vi "DSF.Engine.Memory.Buffer.Insert Channels.Preserve Value.vi"(8 "error in (no error)":errorcluster, 9 "Channel Configuration":T1 {"count" format="%d elements"; "offset" format="%d bytes"}, 10 "VS Channels Array in":dbl[](array[numeric]), 11 "Buffer in":refnum<class "DSF.Engine.Memory.Buffer.lvclass">) -> (0 "error out":errorcluster, 2 "VS Channels Array out":dbl[](array[numeric]), 3 "Buffer out":refnum<class "DSF.Engine.Memory.Buffer.lvclass">)   [LabVIEW 2016, in "DSF.Engine.lvlib" / "DSF.Engine.Memory.Buffer.lvclass"]
uses:
  DSF.Engine.Memory.Buffer.lvclass
  C:/Git/SourceTree/DSF/Source/Submodules/Memory Manager/Source/Classes/Pointer/Memory.Pointer.lvclass
  Typedefs/DSF.Engine.Buffer Channel Configuration.ctl
  Typedefs/DSF.Shared.Data Type.ctl
  Submodules/Memory Manager/Source/Classes/Pointer/Memory.Pointer.lvclass/Memory.Pointer.ctl
  DSF.Engine.Memory.Buffer.Write.1D.Bool.vi
  DSF.Engine.Memory.Buffer.Write.1D.SGL.vi
  DSF.Engine.Memory.Buffer.Write.1D.DBL.vi
  DSF.Engine.Memory.Buffer.Write.1D.I8.vi
  DSF.Engine.Memory.Buffer.Write.1D.I16.vi
  DSF.Engine.Memory.Buffer.Write.1D.I32.vi
  DSF.Engine.Memory.Buffer.Write.1D.I64.vi
  DSF.Engine.Memory.Buffer.Write.1D.U8.vi
  DSF.Engine.Memory.Buffer.Write.1D.U16.vi
  DSF.Engine.Memory.Buffer.Write.1D.U32.vi
  DSF.Engine.Memory.Buffer.Write.1D.U64.vi
  Submodules/Memory Manager/Source/Classes/Pointer/Methods/Memory.Pointer.Write.vi
  Submodules/Memory Manager/Source/Classes/Pointer/Methods/Memory.Pointer.Write.Safe.1D.Bool.vi
  Submodules/Memory Manager/Source/Classes/Pointer/Methods/Memory.Pointer.Write.Safe.1D.SGL.vi
  Submodules/Memory Manager/Source/Classes/Pointer/Methods/Memory.Pointer.Write.Safe.1D.DBL.vi
  Submodules/Memory Manager/Source/Classes/Pointer/Methods/Memory.Pointer.Write.Safe.1D.I8.vi
  Submodules/Memory Manager/Source/Classes/Pointer/Methods/Memory.Pointer.Write.Safe.1D.I16.vi
  Submodules/Memory Manager/Source/Classes/Pointer/Methods/Memory.Pointer.Write.Safe.1D.I32.vi
  Submodules/Memory Manager/Source/Classes/Pointer/Methods/Memory.Pointer.Write.Safe.1D.I64.vi
  Submodules/Memory Manager/Source/Classes/Pointer/Methods/Memory.Pointer.Write.Safe.1D.U8.vi
  Submodules/Memory Manager/Source/Classes/Pointer/Methods/Memory.Pointer.Write.Safe.1D.U16.vi
  Submodules/Memory Manager/Source/Classes/Pointer/Methods/Memory.Pointer.Write.Safe.1D.U32.vi
  Submodules/Memory Manager/Source/Classes/Pointer/Methods/Memory.Pointer.Write.Safe.1D.U64.vi
  Submodules/Memory Manager/Source/Classes/Pointer/Methods/Memory.Pointer.Write.Unsafe.1D.Bool.vi
  Submodules/Memory Manager/Source/Classes/Pointer/Methods/Memory.Pointer.Parameter Check.Null Pointer.vi
  Submodules/Memory Manager/Source/Classes/Pointer/Methods/Memory.Pointer.Parameter Check.Subset.Power of 2.vi
  Submodules/Memory Manager/Source/Classes/Pointer/Methods/Memory.Pointer.Write.Unsafe.1D.SGL.vi
  Submodules/Memory Manager/Source/Classes/Pointer/Methods/Memory.Pointer.Write.Unsafe.1D.DBL.vi
  Submodules/Memory Manager/Source/Classes/Pointer/Methods/Memory.Pointer.Write.Unsafe.1D.I8.vi
  Submodules/Memory Manager/Source/Classes/Pointer/Methods/Memory.Pointer.Write.Unsafe.1D.I16.vi
  Submodules/Memory Manager/Source/Classes/Pointer/Methods/Memory.Pointer.Write.Unsafe.1D.I32.vi
  Submodules/Memory Manager/Source/Classes/Pointer/Methods/Memory.Pointer.Write.Unsafe.1D.I64.vi
  Submodules/Memory Manager/Source/Classes/Pointer/Methods/Memory.Pointer.Write.Unsafe.1D.U8.vi
  Submodules/Memory Manager/Source/Classes/Pointer/Methods/Memory.Pointer.Write.Unsafe.1D.U16.vi
  Submodules/Memory Manager/Source/Classes/Pointer/Methods/Memory.Pointer.Write.Unsafe.1D.U32.vi
  Submodules/Memory Manager/Source/Classes/Pointer/Methods/Memory.Pointer.Write.Unsafe.1D.U64.vi
  Submodules/Memory Manager/Source/Classes/Pointer/Accessors/Get Address.vi
  Submodules/Memory Manager/Source/Classes/Pointer/Methods/Memory.Pointer.Errors.vi
  Submodules/Memory Manager/Source/Classes/Pointer/Methods/Memory.Pointer.Errors.Null Pointer.vi
  Submodules/Memory Manager/Source/Classes/Pointer/Methods/Memory.Pointer.Errors.Out of Bounds.vi
  Submodules/Memory Manager/Source/Classes/Pointer/Accessors/Get Size.vi
  Submodules/Memory Manager/Source/VIs/Memory.Count to Size.Power of 2.vi
  Submodules/Memory Manager/Source/Classes/Pointer/Methods/Memory.Pointer.Errors.Create Error.vi
  Submodules/Memory Manager/Source/Submodules/SEH/Source/VIs/Static Error Handling.Source Buffer.Write.String.vi
  Submodules/Memory Manager/Source/Classes/Pointer/Methods/Memory.Pointer.Errors.Write Pointer Size.vi
  Submodules/Memory Manager/Source/Submodules/SEH/Source/VIs/Static Error Handling.Source Buffer.Write.Numeric.Scalar.Base10.vi
  Submodules/Memory Manager/Source/Submodules/SEH/Source/VIs/Static Error Handling.Source Buffer.Write.Numeric.Scalar.Base10 (U64).vi
  Submodules/Memory Manager/Source/Submodules/SEH/Source/VIs/Static Error Handling.Error Cluster Constant.vi
  Submodules/Memory Manager/Source/Submodules/SEH/Source/VIs/Static Error Handling.Error Cluster Constant (256B).vi
  Submodules/Memory Manager/Source/Submodules/SEH/Source/VIs/Static Error Handling.Parameters.Status.Set.vi
  Submodules/Memory Manager/Source/Submodules/SEH/Source/VIs/Static Error Handling.Parameters.Code.Set.vi
  Submodules/Memory Manager/Source/Submodules/SEH/Source/VIs/Static Error Handling.Parameters.VI Source.Set.vi
  Submodules/Memory Manager/Source/Constants/Memory.Constants.vi
  Submodules/Memory Manager/Source/Constants/Memory.Constants.Library Name.vi
  Submodules/Memory Manager/Source/Classes/Pointer/Methods/Memory.Pointer.Errors.Get Info.vi
  DSF.Shared.lvlib
  DSF.Engine.lvlib
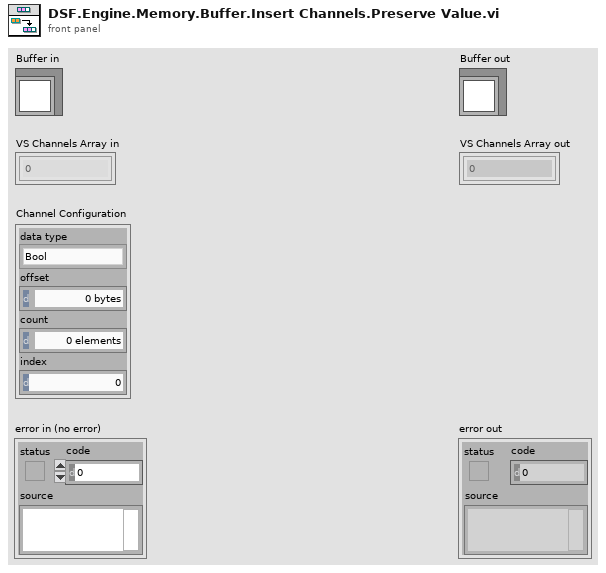
[diagram p1: front panel]
types:
  T1 = typedef "DSF.Engine.lvlib/DSF.Engine.Buffer Channel Configuration.ctl" = cluster{"data type":T2, "offset":u64, "count":u64, "index":u64}
  T2 = typedef "DSF.Shared.lvlib/DSF.Shared.Data Type.ctl" = enum8{"Bool", "SGL", "DBL", "I8", "I16", "I32", "I64", "U8", "U16", "U32", "U64"}
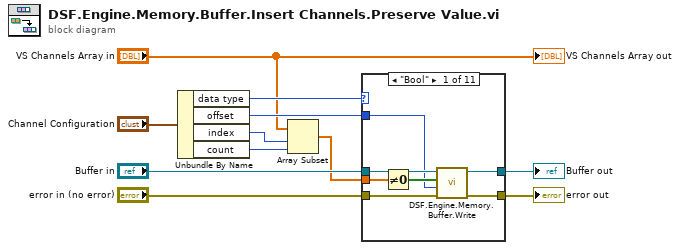
[diagram p0: block diagram]
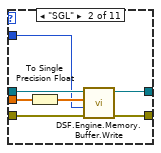
[diagram p2: hidden frame]
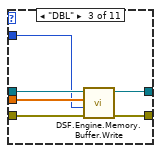
[diagram p3: hidden frame]
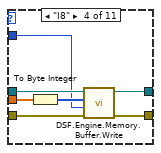
[diagram p4: hidden frame]
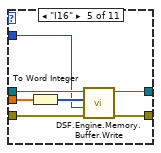
[diagram p5: hidden frame]
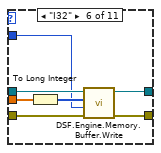
[diagram p6: hidden frame]
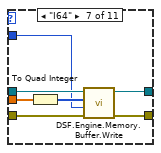
[diagram p7: hidden frame]
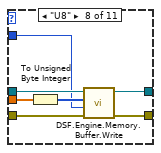
[diagram p8: hidden frame]
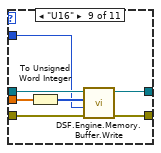
[diagram p9: hidden frame]
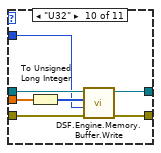
[diagram p10: hidden frame]
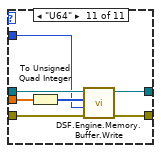
[diagram p11: hidden frame]
diagram:
  n1 = Unbundle By Name("Channel Configuration") -> ("data type"=w5:T2, "offset"=w11:u64, "index"=w9:u64, "count"=w8:u64)
  n2 = Array Subset(array="VS Channels Array in", index=w9, length=w8) -> (w2:dbl[])
  n3 = case shown="\"Bool\"" w5 {
    tunnel: "Buffer in" -> [w18 w25 w31 w38 w45 w52 w59 w66 w73 w80 w87]
    tunnel: w2 -> [w13 w20 w27 w33 w40 w47 w54 w61 w68 w75 w82]
    tunnel: "error in (no error)" -> [w17 w24 w30 w37 w44 w51 w58 w65 w72 w79 w86]
    tunnel: [w16 w23 w29 w36 w43 w50 w57 w64 w71 w78 w85] -> w6
    tunnel: w11 -> [w14 w21 w26 w34 w41 w48 w55 w62 w69 w76 w83]
    tunnel: [w12 w19 w28 w32 w39 w46 w53 w60 w67 w74 w81] -> w3
    frame "Bool" {
      n4 = Not Equal To 0?(x=w13) -> (x != 0?=w15:bool[])
      n5 = call-poly "DSF.Engine.Memory.Buffer.Write.vi"("error in (no error)"=w17, "offset (0)"=w14, "buffer in"=w15, "Buffer in"=w18) -> ("error out"=w16:errorcluster, "Buffer out"=w12:refnum<class "DSF.Engine.Memory.Buffer.lvclass">)  [unwired: 4 in, 2 out]
    }
    frame "SGL" {
      n6 = To Single Precision Float(number=w20) -> (single precision float=w22:sgl[])
      n7 = call-poly "DSF.Engine.Memory.Buffer.Write.vi"("error in (no error)"=w24, "offset (0)"=w21, "buffer in"=w22, "Buffer in"=w25) -> ("error out"=w23:errorcluster, "Buffer out"=w19:refnum<class "DSF.Engine.Memory.Buffer.lvclass">)  [unwired: 4 in, 2 out]
    }
    frame "DBL" {
      n8 = call-poly "DSF.Engine.Memory.Buffer.Write.vi"("error in (no error)"=w30, "offset (0)"=w26, "buffer in"=w27, "Buffer in"=w31) -> ("error out"=w29:errorcluster, "Buffer out"=w28:refnum<class "DSF.Engine.Memory.Buffer.lvclass">)  [unwired: 4 in, 2 out]
    }
    frame "I8" {
      n9 = To Byte Integer(number=w33) -> (8bit integer=w35:i8[])
      n10 = call-poly "DSF.Engine.Memory.Buffer.Write.vi"("error in (no error)"=w37, "offset (0)"=w34, "buffer in"=w35, "Buffer in"=w38) -> ("error out"=w36:errorcluster, "Buffer out"=w32:refnum<class "DSF.Engine.Memory.Buffer.lvclass">)  [unwired: 4 in, 2 out]
    }
    frame "I16" {
      n11 = To Word Integer(number=w40) -> (16bit integer=w42:i16[])
      n12 = call-poly "DSF.Engine.Memory.Buffer.Write.vi"("error in (no error)"=w44, "offset (0)"=w41, "buffer in"=w42, "Buffer in"=w45) -> ("error out"=w43:errorcluster, "Buffer out"=w39:refnum<class "DSF.Engine.Memory.Buffer.lvclass">)  [unwired: 4 in, 2 out]
    }
    frame "I32" {
      n13 = To Long Integer(number=w47) -> (32bit integer=w49:i32[])
      n14 = call-poly "DSF.Engine.Memory.Buffer.Write.vi"("error in (no error)"=w51, "offset (0)"=w48, "buffer in"=w49, "Buffer in"=w52) -> ("error out"=w50:errorcluster, "Buffer out"=w46:refnum<class "DSF.Engine.Memory.Buffer.lvclass">)  [unwired: 4 in, 2 out]
    }
    frame "I64" {
      n15 = To Quad Integer(1:w54) -> (0:w56:i64[])
      n16 = call-poly "DSF.Engine.Memory.Buffer.Write.vi"("error in (no error)"=w58, "offset (0)"=w55, "buffer in"=w56, "Buffer in"=w59) -> ("error out"=w57:errorcluster, "Buffer out"=w53:refnum<class "DSF.Engine.Memory.Buffer.lvclass">)  [unwired: 4 in, 2 out]
    }
    frame "U8" {
      n17 = To Unsigned Byte Integer(number=w61) -> (unsigned 8bit integer=w63:u8[])
      n18 = call-poly "DSF.Engine.Memory.Buffer.Write.vi"("error in (no error)"=w65, "offset (0)"=w62, "buffer in"=w63, "Buffer in"=w66) -> ("error out"=w64:errorcluster, "Buffer out"=w60:refnum<class "DSF.Engine.Memory.Buffer.lvclass">)  [unwired: 4 in, 2 out]
    }
    frame "U16" {
      n19 = To Unsigned Word Integer(number=w68) -> (unsigned 16bit integer=w70:u16[])
      n20 = call-poly "DSF.Engine.Memory.Buffer.Write.vi"("error in (no error)"=w72, "offset (0)"=w69, "buffer in"=w70, "Buffer in"=w73) -> ("error out"=w71:errorcluster, "Buffer out"=w67:refnum<class "DSF.Engine.Memory.Buffer.lvclass">)  [unwired: 4 in, 2 out]
    }
    frame "U32" {
      n21 = To Unsigned Long Integer(number=w75) -> (unsigned 32bit integer=w77:u32[])
      n22 = call-poly "DSF.Engine.Memory.Buffer.Write.vi"("error in (no error)"=w79, "offset (0)"=w76, "buffer in"=w77, "Buffer in"=w80) -> ("error out"=w78:errorcluster, "Buffer out"=w74:refnum<class "DSF.Engine.Memory.Buffer.lvclass">)  [unwired: 4 in, 2 out]
    }
    frame "U64" {
      n23 = To Unsigned Quad Integer(1:w82) -> (0:w84:u64[])
      n24 = call-poly "DSF.Engine.Memory.Buffer.Write.vi"("error in (no error)"=w86, "offset (0)"=w83, "buffer in"=w84, "Buffer in"=w87) -> ("error out"=w85:errorcluster, "Buffer out"=w81:refnum<class "DSF.Engine.Memory.Buffer.lvclass">)  [unwired: 4 in, 2 out]
    }
  }
  "error out" <- w6
  "Buffer out" <- w3
  "VS Channels Array out" <- "VS Channels Array in"
